vi "16-ParseLiteral.vi"(11 "BITS in":bool[](array[boolean])) -> (2 "Value":u64, 3 "BITS out":bool[](array[boolean]))   [LabVIEW 2019, in "16.lvlib"]
uses:
  16.lvlib
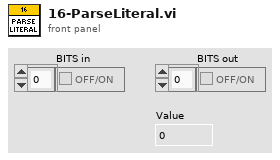
[diagram p1: front panel]
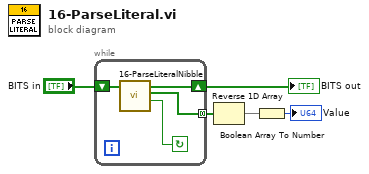
[diagram p0: block diagram]
diagram:
  n1 = while {
    shift-right: [w8] -> w5
    shift-left: "BITS in" -> [w9]
    tunnel: [w6] -> w3 mode=concatenating
    stop <- w7 continue-if-true
    n2 = call "16-ParseLiteralNibble.vi"("BITS in in"=w9) -> ("Last Nibble?"=w7:bool, "Nibble"=w6:bool[], "BITS out"=w8:bool[])  [unwired: 8 in]
  }
  "BITS out" <- w5
  n3 = Reverse 1D Array(array=w3) -> (reversed array=w2:bool[])
  n4 = Boolean Array To Number(Boolean array=w2) -> (number=→"Value":u64)
